vi "test String to U8_3.vi"(11 "Test Case In":refnum<class "test Electronic Datasheet.lvclass">) -> (0 "error out":errorcluster, 3 "Test Case Out":refnum<class "test Electronic Datasheet.lvclass">)   [LabVIEW 2024, in "test Electronic Datasheet.lvclass"]
uses:
  test Electronic Datasheet.lvclass
  test Electronic Datasheet.lvclass/test Electronic Datasheet.ctl
  Core/Electronic Datasheet.lvlib
  896e62fd-c0ef-4146-ba1f-33cd0e9e8722.vi
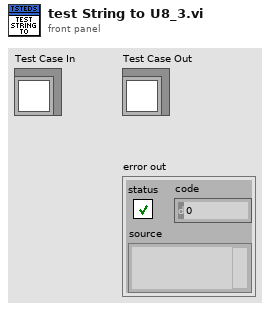
[diagram p1: front panel]
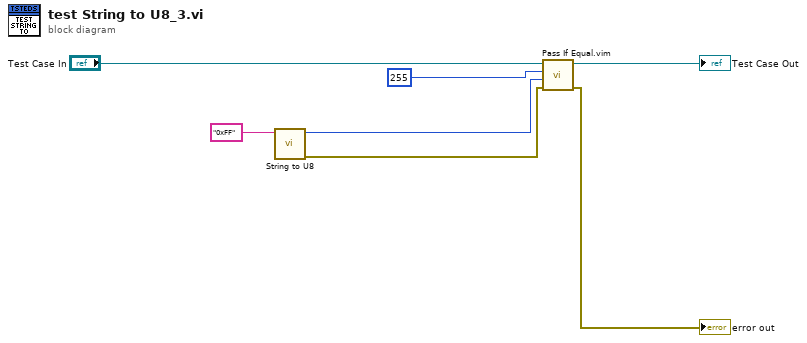
[diagram p0: block diagram]
diagram:
  n1 = call "String to U8.vi"("Integer String"="0xFF" ("String")) -> ("error out"=w3:errorcluster, "U8"=w2:u8)  [unwired: 9 in]
  n2 = call "Pass If Equal.vim"("error in (no error)"=w3, "Actual"=w2, "Expected"=u8 255, "LUnit Test Case In"="Test Case In") -> ("error out"=→"error out":errorcluster, "LUnit Test Case Out"=→"Test Case Out":refnum<class "test Electronic Datasheet.lvclass">)  [unwired: 6 in]
